vi "Apply Flags.vi"(8 "error in (no error)":errorcluster, 10 "FIFO Flags":u64, 11 "CIFChannels in":refnum<class "CIFChannels.lvclass">) -> (0 "error out":errorcluster, 3 "CIFChannels out":refnum<class "CIFChannels.lvclass">)   [LabVIEW 2021, in "CIFChannels.lvclass"]
uses:
  CIFChannels.lvclass
  CIFChannels.lvclass/CIFChannels.ctl
  ChannelCommon/ChannelCommon.lvlib
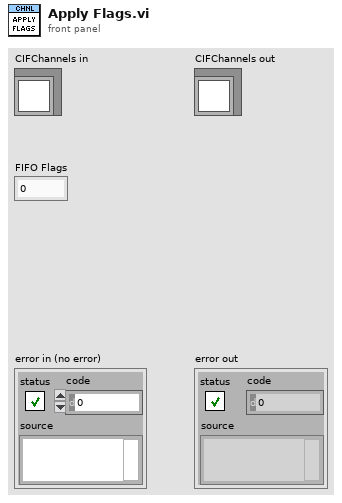
[diagram p1: front panel]
types:
  T1 = typedef "ChannelCommon.lvlib/FIFO Flags.ctl" = cluster{"Backpressure":bool}
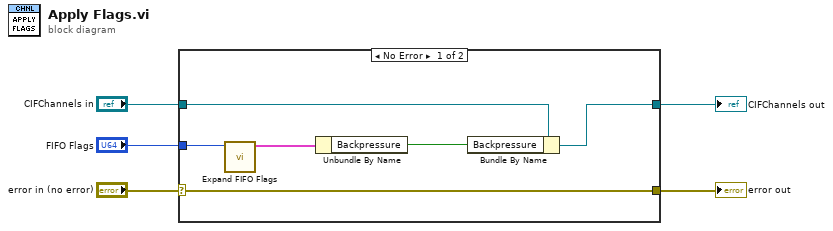
[diagram p0: block diagram]
diagram:
  n1 = case shown="No Error" "error in (no error)" {
    selector: "error in (no error)" -> [w11 w13]
    tunnel: [w11 w13] -> w4
    tunnel: [w6 w12] -> w2
    tunnel: "CIFChannels in" -> [w8 w12]
    tunnel: "FIFO Flags" -> [w9 _]
    frame No Error {
      n2 = call "Expand FIFO Flags.vi"("FIFO Flags"=w9) -> ("Flags"=w10:T1)  [unwired: 10 in]
      n3 = Unbundle By Name(w10) -> ("Backpressure"=w7:bool)
      n4 = Bundle By Name(cluster=w8, "Backpressure"=w7) -> (w6:refnum<class "CIFChannels.lvclass">)
    }
    frame Error {
    }
  }
  "error out" <- w4
  "CIFChannels out" <- w2
